vi "test_livefeed.vi"() -> ()   [LabVIEW 2021]
uses:
  <vilib>/userDefined/High Color/IMAQdx.ctl
  <vilib>/vision/driver/NI_Vision_Acquisition_Software.lvlib
panel:
  out "Buffer Number Out":u32
  out "error out":errorcluster
  in  "Device":T1="cam1"
  out "Time":u32
  out "Image viewer":T2(plugin-control)
  in  "stop":bool
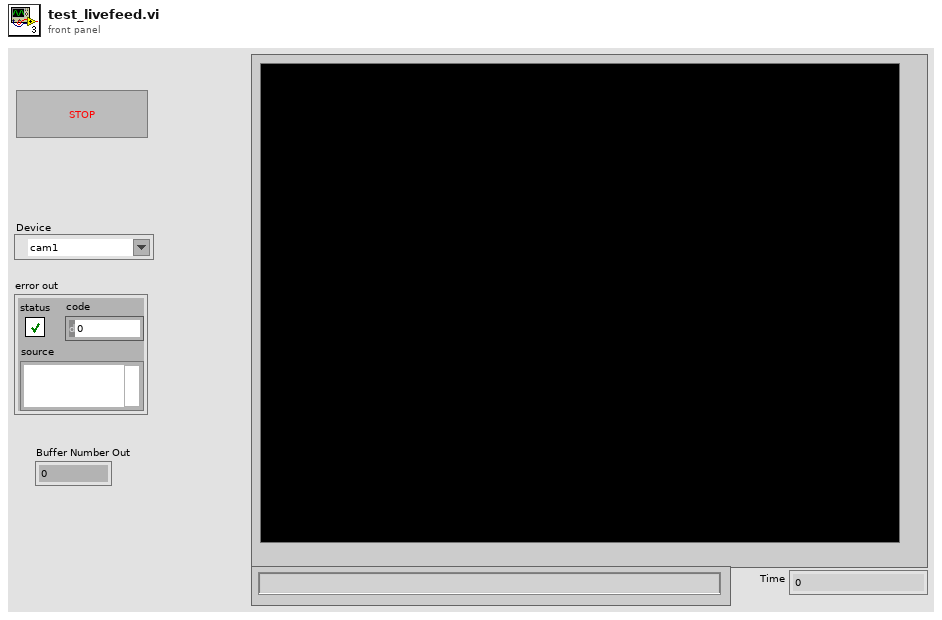
[diagram p1: front panel]
types:
  T1 = typedef "IMAQdx.ctl" = refnum<k21>
  T2 = typedef "IMAQ Image.ctl" = refnum<image>
  T3 = typedef "Image Type" = u32
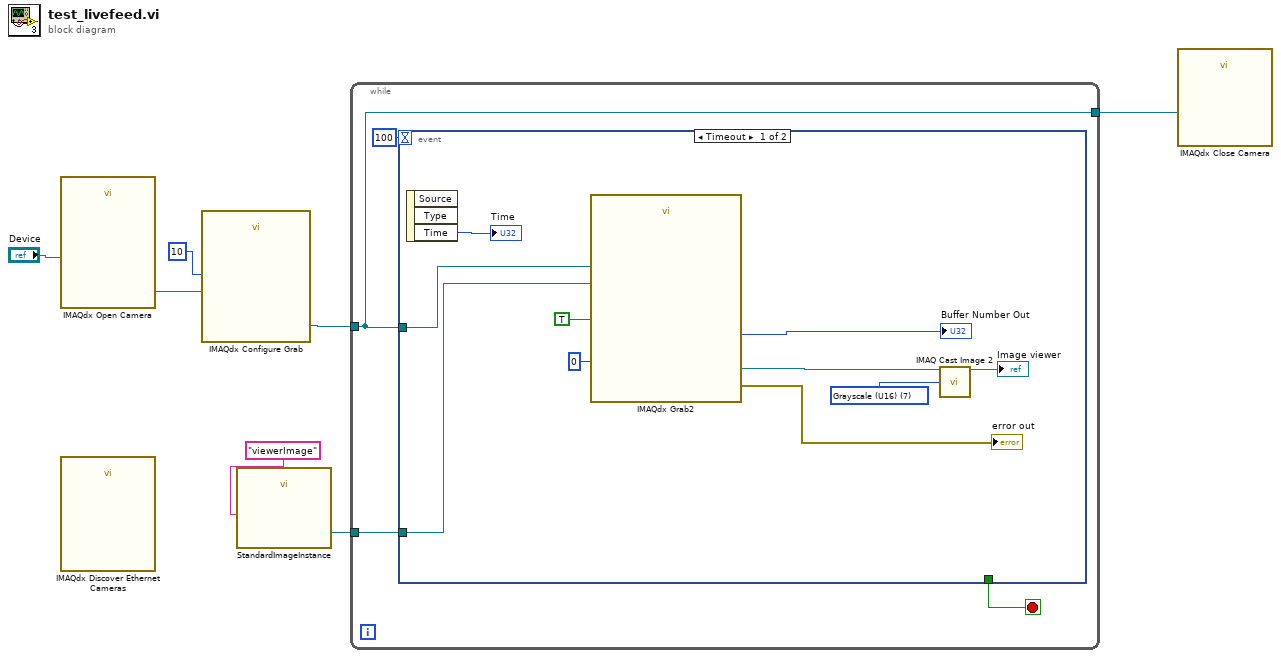
[diagram p0: block diagram]
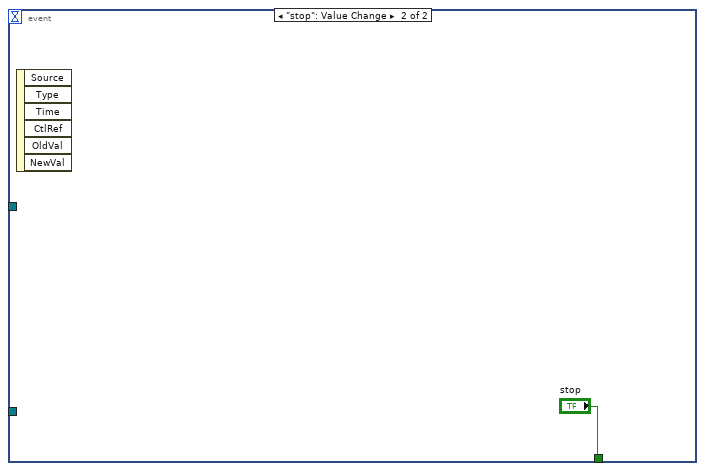
[diagram p2: hidden frame]
diagram:
  n1 = call <vilib>:"IMAQdx Open Camera.vi"("Session In"="Device") -> ("Session Out"=w4:T1)  [unwired: 9 in, 1 out]
  n2 = call <vilib>:"IMAQdx Discover Ethernet Cameras.vi"() -> ()  [unwired: 11 in, 1 out]
  n3 = call <vilib>:"IMAQdx Configure Grab.vi"("Number of Buffers"=u32 10, "Session In"=w4) -> ("Session Out"=w3:T1)  [unwired: 8 in, 1 out]
  n4 = call "StandardImageInstance.vi"("Image Name"="viewerImage") -> ("Refnum out"=w1:T2)  [unwired: 10 in]
  n5 = while {
    tunnel: w3 -> [w10]
    tunnel: [w10] -> w5
    tunnel: w1 -> [w8]
    stop <- w9 stop-if-true
    n6 = event shown="[0] Timeout" {
      selector: _ -> [_ _]
      dyn-events: _ -> [_ _]
      timeout: 100 -> [_ _]
      tunnel: [_ "stop"] -> w9
      tunnel: w10 -> [w17 _]
      tunnel: w8 -> [w12 _]
      event Timeout {
        w20 = T3 7 items=["Grayscale (U8)", "Grayscale (I16)", "Grayscale (SGL)", "Complex (CSG)", "RGB (U32)", "HSL (U32)", "RGB (U64)", "Grayscale (U16)"] ("Image Type")
        n7 = event-data() -> ("Time"=→"Time":u32)  [unwired: 1 in, 2 out]
        n8 = call <vilib>:"IMAQdx Grab2.vi"("Timeout (ms)"=0, "Wait for Next Buffer? (Yes)"=TRUE, "Image In"=w12, "Session In"=w17) -> ("error out"=→"error out":errorcluster, "Buffer Number Out"=→"Buffer Number Out":u32, "Image Out"=w21:T2)  [unwired: 4 in, 1 out]
        n9 = call "IMAQ Cast Image 2"("Image Src"=w21, "Image Type"=w20) -> ("Image Dst Out"=→"Image viewer":T2)  [unwired: 12 in, 1 out]
      }
      event "stop": Value Change {
        n10 = event-data() -> ()  [unwired: 1 in, 6 out]
      }
    }
  }
  n11 = call <vilib>:"IMAQdx Close Camera.vi"("Session In"=w5) -> ()  [unwired: 10 in, 1 out]
